vi "PH_Beamline.set GUI elements.vi"(0 "i ref in":refnum<vi>, 1 "Vision Knobs":refnum<vi>[](array[refnum]), 2 "Vision on this node?":bool, 5 "error in (no error)":errorcluster) -> (14 "i ref out":refnum<vi>, 19 "error out":errorcluster)   [LabVIEW 2014, in "PH_Beamline.lvlib"]
doc: "Within this VI GUI elements are set."
uses:
  PH_Beamline.lvlib
  PH_BL-Master/PH_BL-Master.lvlib
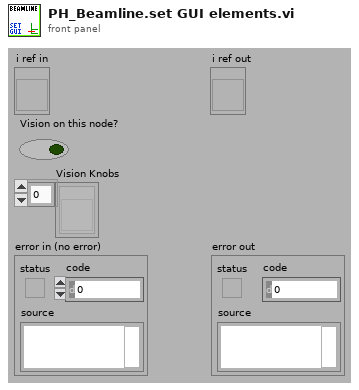
[diagram p1: front panel]
types:
  T1 = typedef "PH_BL-Master.lvlib/PH_BL-Master.i attribute.ctl" = cluster{"Remote controlled":bool, "Boolean Condition Service Subscriber":refnum<vi>[], "Picture Condition Service Subscriber":refnum<vi>[], "R2S":cluster{"GUI Ref":refnum<vi>, "State":bool}, "Vacua":cluster{"GUI Ref":refnum<vi>, "Limit":dbl, "Curr Value":dbl, "in range":bool}[], "O2 Inspection":cluster{"GUI Ref":refnum<vi>, "Concentration":dbl, "State":T2}[], "Boolean Status Service Subscriber":cluster{"GUI Ref":refnum<vi>, "Status":T2, "no Link?":bool, "Status Subscriber Class":T3}[], "Picture Status Service Subscriber":cluster{"GUI Ref":refnum<vi>, "Status":T2, "no Link?":bool, "Status Subscriber Class":T3}[], "6P 4Q Service Subscriber":cluster{"GUI Ref":refnum<vi>, "Selector":T4, "no Link?":bool}[], "Index of latest 6P 4Q changing Instance":i32, "Index of latest Picture Status changing Instance":i32, "Index of latest Boolean Status changing Instance":i32, "Vision ID on same Node":string, "Start Phase over?":bool, "GUI Ref Delete":refnum<vi>}
  T2 = typedef "PH_StatusHandler.lvlib/PH_StatusHandler.Status.ctl" = i16
  T3 = typedef "PH_BL-Master.lvlib/PH_BL-Master.Status Subscriber Class.ctl" = enum16{"unknown", "Switch", "BB", "6P Switch", "Switch GUI", "Switch and 6P State", "Force Sensor"}
  T4 = typedef "PH_4_Pos_Selector.lvlib/PH_4_Pos_Selector.Position Selector.ctl" = u16
  T5 = cluster{"GUI Ref":refnum<vi>, "Selector":T4, "no Link?":bool}[]
  T6 = cluster{"GUI Ref":refnum<vi>, "Status":T2, "no Link?":bool, "Status Subscriber Class":T3}[]
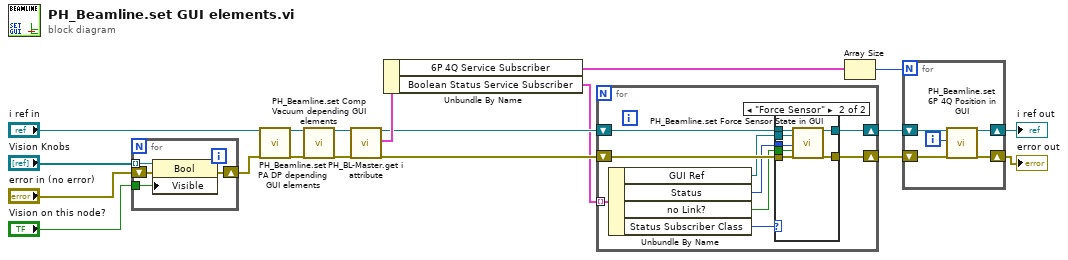
[diagram p0: block diagram]
diagram:
  n1 = for {
    shift-right: [w23] -> w13
    shift-left: "error in (no error)" -> [w21]
    tunnel: "Vision on this node?" -> [w22]
    tunnel: "Vision Knobs" -> [w20] mode=indexing
    n2 = property class="Bool"(reference=w20, error in=w21, "Visible"=w22) -> (error out=w23:errorcluster)  [unwired: 1 out]
  }
  n3 = call "PH_Beamline.set PA DP depending GUI elements.vi"("VI in"="i ref in", "error in (no error)"=w13) -> ("VI out"=w17:refnum<vi>, "error out"=w18:errorcluster)  [unwired: 16 in]
  n4 = call "PH_Beamline.set Comp Vacuum depending GUI elements.vi"("VI in"=w17, "error in (no error)"=w18) -> ("VI out"=w11:refnum<vi>, "error out"=w12:errorcluster)  [unwired: 16 in]
  n5 = call "PH_BL-Master.get i attribute.vi"("i ref in"=w11, "error in (no error)"=w12) -> ("i ref out"=w3:refnum<vi>, "i attribute"=w10:T1, "error out"=w5:errorcluster)  [unwired: 15 in]
  n6 = Unbundle By Name(w10) -> ("6P 4Q Service Subscriber"=w7:T5, "Boolean Status Service Subscriber"=w1:T6)
  n7 = for {
    shift-right: [w31] -> w4
    shift-left: w5 -> [w32]
    shift-right: [w29] -> w2
    shift-left: w3 -> [w30]
    tunnel: w1 -> [w28] mode=indexing
    n8 = Unbundle By Name(w28) -> ("GUI Ref"=w27:refnum<vi>, "Status"=w26:T2, "no Link?"=w25:bool, "Status Subscriber Class"=w24:T3)
    n9 = case shown="\"Force Sensor\"" w24 {
      tunnel: w32 -> [w33 w41]
      tunnel: [w33 w40] -> w31
      tunnel: w30 -> [w34 w39]
      tunnel: [w34 w38] -> w29
      tunnel: w27 -> [_ w37]
      tunnel: w26 -> [_ w36]
      tunnel: w25 -> [_ w35]
      frame Default {
      }
      frame "Force Sensor" {
        n10 = call "PH_Beamline.set Force Sensor State in GUI.vi"("i ref in"=w39, "Force Sensor GUI Ref"=w37, "Subscriber State"=w36, "No Link"=w35, "error in (no error)"=w41) -> ("i ref out"=w38:refnum<vi>, "error out"=w40:errorcluster)  [unwired: 13 in]
      }
    }
  }
  n11 = Array Size(array=w7) -> (size(s)=w6:i32)
  n12 = for {
    N: w6 -> [_]
    shift-right: [w45] -> w9
    shift-left: w2 -> [w46]
    shift-right: [w43] -> w8
    shift-left: w4 -> [w44]
    i -> [w42]
    n13 = call "PH_Beamline.set 6P 4Q Position in GUI.vi"("VI in"=w46, "Index 6P 4Q Instance to change"=w42, "error in (no error)"=w44) -> ("VI out"=w45:refnum<vi>, "error out"=w43:errorcluster)  [unwired: 15 in]
  }
  "i ref out" <- w9
  "error out" <- w8
